vi "SignalGenerator.vi"(9 "Amplitude":dbl, 10 "Frequency":dbl) -> ()   [LabVIEW 2014]
panel:
  out "error out":errorcluster
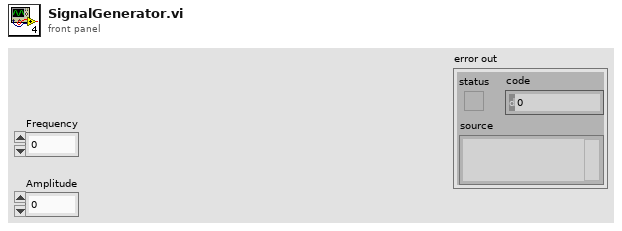
[diagram p1: front panel]
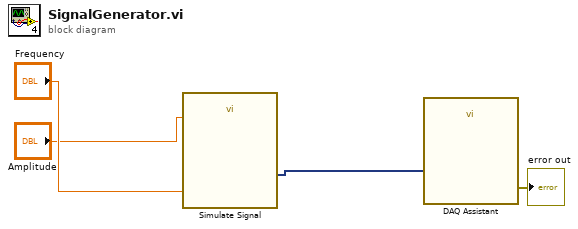
[diagram p0: block diagram]
diagram:
  n1 = call "Simulate Signal"("Frequency"="Frequency", "Amplitude"="Amplitude") -> ("Sine"=w2:dynamicdata)  [unwired: 12 in, 1 out]
  n2 = call "DAQ Assistant"("data"=w2) -> ("error out"=→"error out":errorcluster)  [unwired: 16 in, 2 out]
